vi "ROS_Topic_Write.vi"(3 "error in (no error)":errorcluster, 4 "Msg in":string, 5 "ROS in":T1={"topic port"=0, "Node"="", "topic"="", "type"="", "node port"=0, "error "={"status"=FALSE, "code"=0, "source"=""}, "Direction"=enum."Node", "Update (ms)"=1, "queue size"=1}) -> (0 "error out":errorcluster, 2 "ROS out":T1={"topic port"=0, "Node"="", "topic"="", "type"="", "node port"=0, "error "={"status"=FALSE, "code"=0, "source"=""}, "Direction"=enum."Node", "Update (ms)"=1, "queue size"=1})   [LabVIEW 2012]
doc: "Prepends the length to Msg in before sending out the data on the specified topic. Use only for publishers and service clients. Messages need to be formatted using Message Building functionality. \n\nSetting Continuous to True will instruct the server to publish the message it received as quickly as possible, updating the message when a new ROS_Topic_Write is called."
uses:
  <userlib>/ROSforLV/ROS/Code/SubVIs/_ROSControl.ctl
  <userlib>/ROSforLV/ROS/Code/SubVIs/_ROSDirection.ctl
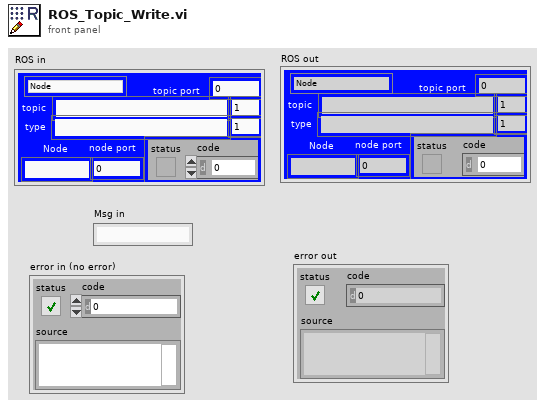
[diagram p1: front panel]
types:
  T1 = typedef "_ROSControl.ctl" = cluster{"topic port":u16, "Node":string, "topic":string, "type":string, "node port":u16, "error ":errorcluster, "Direction":T2, "Update (ms)":u16, "queue size":u16}
  T2 = typedef "_ROSDirection.ctl" = enum16{"Node", "Publisher", "Subscriber", "Service Client"}
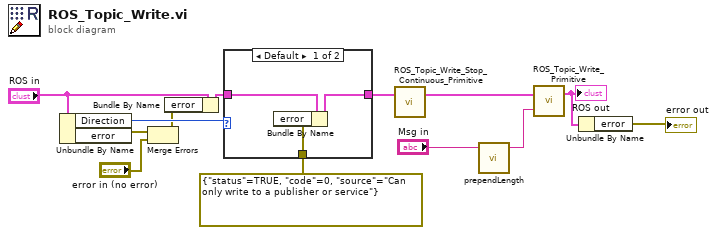
[diagram p0: block diagram]
diagram:
  n1 = Unbundle By Name("ROS in") -> ("Direction"=w9:T2, "error"=w8:errorcluster)
  n2 = Merge Errors(w8, "error in (no error)") -> (w5:errorcluster)
  n3 = Bundle By Name(cluster="ROS in", "error"=w5) -> (w6:T1)
  n4 = case shown="Default" w9 {
    tunnel: [w15 w17] -> w11
    tunnel: w6 -> [w14 w17]
    tunnel: errorcluster {"status"=TRUE, "code"=0, "source"="Can only write to a publisher or service"} ("error out") -> [w16 _]
    frame Default {
      n5 = Bundle By Name(cluster=w14, "error"=w16) -> (w15:T1)
    }
    frame "Publisher", "Service Client" {
    }
  }
  n6 = call <userlib>:"ROS_Topic_Write_Stop_Continuous_Primitive.vi"("ROS in"=w11) -> ("ROS out"=w3:T1)  [unwired: 2 in]
  n7 = call <userlib>:"prependLength.vi"("msg in"="Msg in") -> ("msg out"=w12:string)  [unwired: 4 in]
  n8 = call <userlib>:"ROS_Topic_Write_Primitive.vi"("Msg in"=w12, "ROS in"=w3) -> ("ROS out"=w1:T1)  [unwired: 1 in]
  "ROS out" <- w1
  n9 = Unbundle By Name(w1) -> ("error"=→"error out":errorcluster)
